vi "Get Frame Configuration.vi"(8 "error in":errorcluster, 11 "Parent Ref":T4=18446744073709551615 format="%.0x") -> (0 "error out":errorcluster, 2 "Selected Channels":T1 {"CRC"."Data Type" items=["Signed", "Unsigned", "IEEE Float"]; "Rolling Counter"."Data Type" items=["Signed", "Unsigned", "IEEE Float"]; "Input Channels"."Data Type" items=["Signed", "Unsigned", "IEEE Float"]}, 3 "Parent Ref Out":T4=18446744073709551615 format="%.0x")   [LabVIEW 2015, in "Protection and Rolling Counter Addon Shared.lvlib"]
uses:
  Protection and Rolling Counter Addon Shared.lvlib
  <vilib>/NI Veristand/Custom Device API/Custom Device Item Ref.ctl
  Types/FrameConfiguration.ctl
  Types/InputChannelConfiguration.ctl
  Types/Protection Type.ctl
  GUID Lookup.vi
  <vilib>/NI Veristand/Custom Device API/Get Item Property (Variant).vi
  <vilib>/NI Veristand/Custom Device API/Custom Device API.lvlib
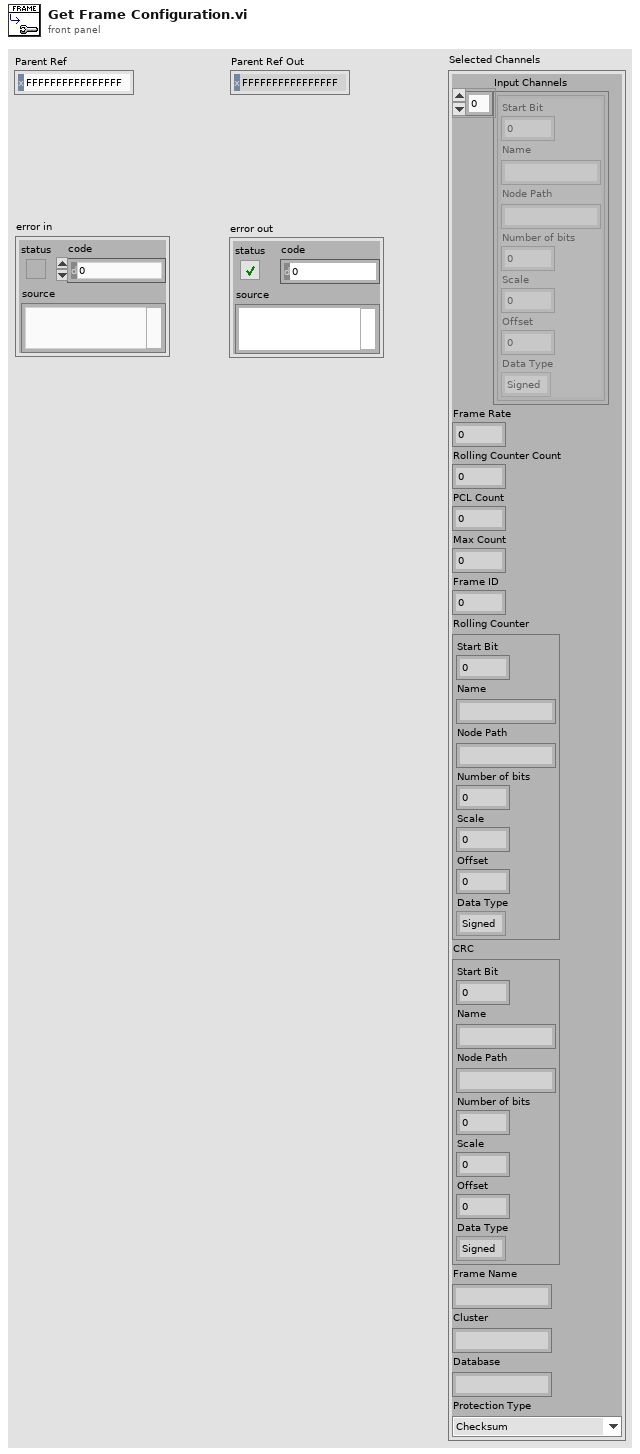
[diagram p1: front panel]
types:
  T1 = typedef "Protection and Rolling Counter Addon Shared.lvlib/FrameConfiguration.ctl" = cluster{"Input Channels":T2[], "Frame Rate":dbl, "Rolling Counter Count":dbl, "PCL Count":u64, "Max Count":dbl, "Frame ID":u32, "Rolling Counter":T2, "CRC":T2, "Frame Name":string, "Cluster":string, "Database":string, "Protection Type":T3}
  T2 = typedef "Protection and Rolling Counter Addon Shared.lvlib/InputChannelConfiguration.ctl" = cluster{"Start Bit":i32, "Name":string, "Node Path":string, "Number of bits":i32, "Scale":dbl, "Offset":dbl, "Data Type":u32}
  T3 = typedef "Protection and Rolling Counter Addon Shared.lvlib/Protection Type.ctl" = enum16{"Checksum", "CRC", "None (Counter Only)", "CGEA Checksum"}
  T4 = typedef "Custom Device API.lvlib/Custom Device Item Ref.ctl" = u64
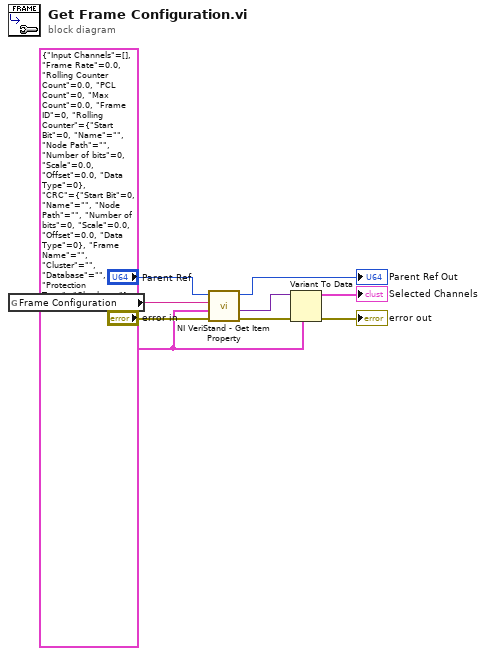
[diagram p0: block diagram]
diagram:
  w1 = T1 {"Input Channels"=[], "Frame Rate"=0.0, "Rolling Counter Count"=0.0, "PCL Count"=0, "Max Count"=0.0, "Frame ID"=0, "Rolling Counter"={"Start Bit"=0, "Name"="", "Node Path"="", "Number of bits"=0, "Scale"=0.0, "Offset"=0.0, "Data Type"=0}, "CRC"={"Start Bit"=0, "Name"="", "Node Path"="", "Number of bits"=0, "Scale"=0.0, "Offset"=0.0, "Data Type"=0}, "Frame Name"="", "Cluster"="", "Database"="", "Protection Type"=enum."Checksum"} ("Selected Channels")
  n1 = global read "GUID Lookup.vi" "Frame Configuration"() -> (w5:string)
  n2 = call-poly <vilib>:"NI VeriStand - Get Item Property.vi"("error in (no error)"="error in", "Default Value"=w1, "Property Name"=w5, "Item Ref in"="Parent Ref") -> ("error out"=w8:errorcluster, "Value"=w3:variant, "Item Ref out"=→"Parent Ref Out":T4)  [unwired: 4 in, 1 out]
  n3 = Variant To Data(error in=w8, type=w1, Variant=w3) -> (data=→"Selected Channels":T1, error out=→"error out":errorcluster)
